vi "Normalize End Of Line.vi"(4 "end of line (Native)":T1(ring), 7 "string in":string) -> (2 "string out":string)   [LabVIEW 2020]
doc: "Converts the line endings of the input string to the line ending format you specify. If you do not specify a line ending format, this VI converts the line endings of the string to the line endings that the current platform expects. Use this VI to make your strings readable by different platforms or by the command line of the current platform."
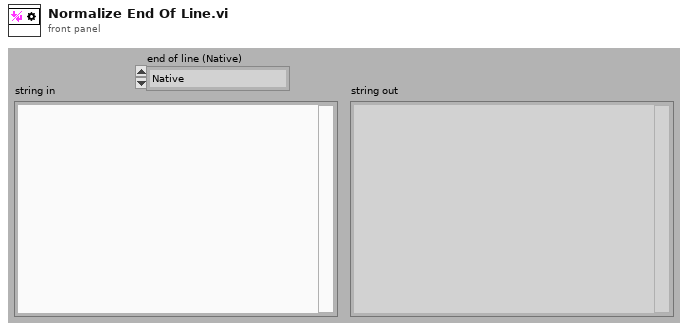
[diagram p1: front panel]
types:
  T1 = enum16{"Native", "Native Command Line", "UNIX", "Macintosh", "DOS"}
  T2 = enum32{"invalid OS target", "Mac OS", "Windows 3.1", "Windows 95/NT", "Solaris 1", "Solaris 2", "HP-UX", "PowerMAX", "Linux", "Irix", "Rhapsody", "BeOS", "AIX", "OSF1", "VxWorks", "PharLap", "Carbon"}
  T3 = enum32{"invalid OS target", "Mac OS", "Windows 3.1", "Windows 95/NT", "Solaris 1", "Solaris 2", "HP-UX", "PowerMAX", "Linux", "Irix", "Rhapsody", "BeOS", "AIX", "OSF1", "VxWorks", "PharLap", "Carbon", "RTX", "Windows x64", "Linux x64", "Mac OS X x64"}
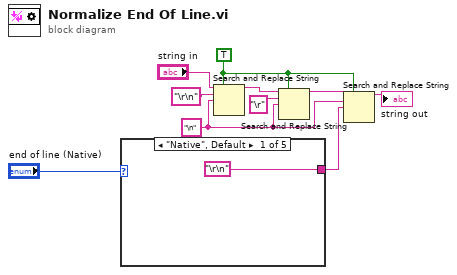
[diagram p0: block diagram]
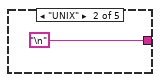
[diagram p2: hidden frame]
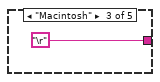
[diagram p3: hidden frame]
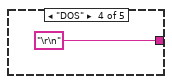
[diagram p4: hidden frame]
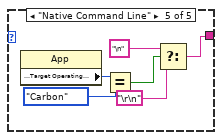
[diagram p5: hidden frame]
diagram:
  w3 = "\n" ("search string")
  w4 = TRUE ("replace all? (F)")
  n1 = case shown="\"Native\", Default" "end of line (Native)" {
    tunnel: ["\r\n" "\n" "\r" "\r\n" w15] -> w2
    frame "Native", Default {
    }
    frame "UNIX" {
    }
    frame "Macintosh" {
    }
    frame "DOS" {
    }
    frame "Native Command Line" {
      n2 = property class="App"() -> ("Application:Target Operating System"=w20:T3)  [unwired: 2 in, 2 out]
      n3 = Equal?(x=w20, y=T2."Carbon" ("Application:Target Operating System")) -> (x = y?=w18:bool)
      n4 = Select(t="\n" ("search string"), s=w18, f="\r\n") -> (s? t:f=w15:string)
    }
  }
  n5 = Search and Replace String(replace all?=w4, input string="string in", search string="\r\n", replace string=w3) -> (result string=w8:string)  [unwired: 4 in, 3 out]
  n6 = Search and Replace String(replace all?=w4, input string=w8, search string="\r", replace string=w3) -> (result string=w5:string)  [unwired: 4 in, 3 out]
  n7 = Search and Replace String(replace all?=w4, input string=w5, search string=w3, replace string=w2) -> (result string=→"string out":string)  [unwired: 4 in, 3 out]
